vi "detencion.vi"(7 "This VI":refnum<vi>, 8 "error in (no error)":errorcluster, 9 "Air flow":refnum<vi>, 10 "Water flow":refnum<vi>) -> (0 "error out":errorcluster)   [LabVIEW 2013]
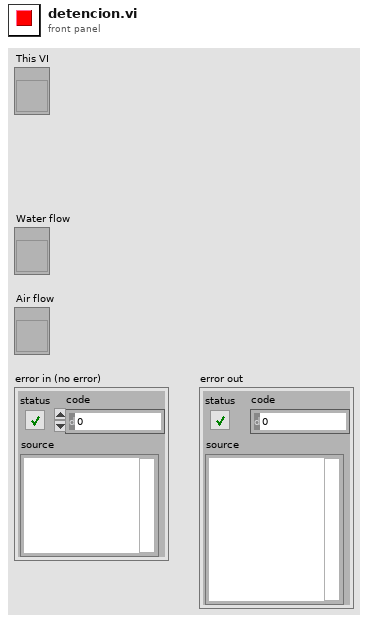
[diagram p1: front panel]
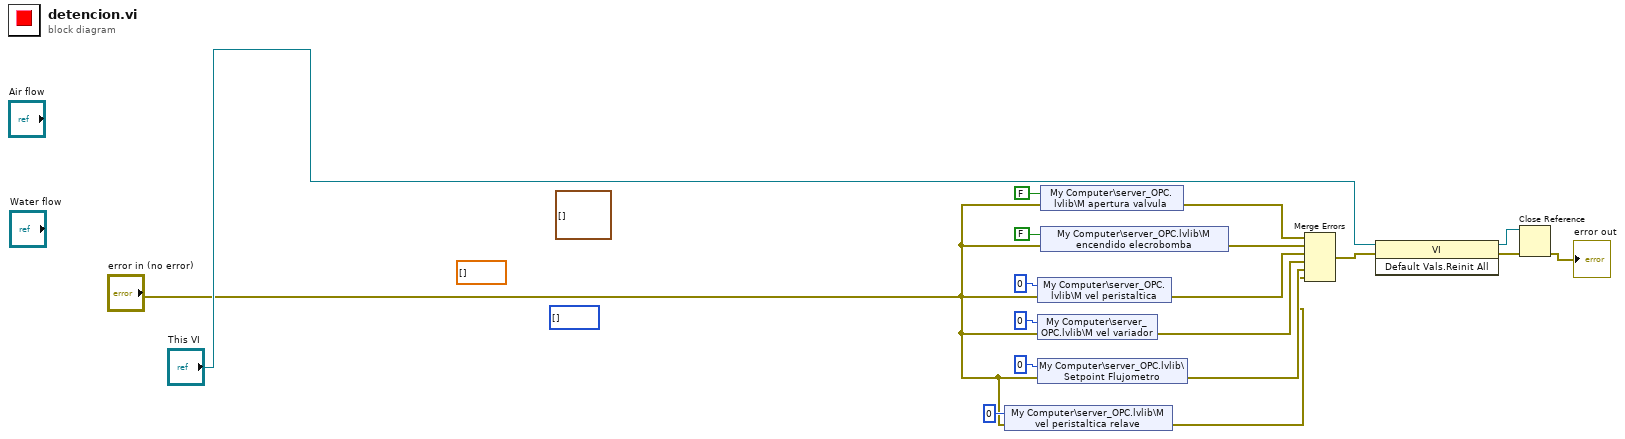
[diagram p0: block diagram]
diagram:
  (unwired) cluster{"pulp flow":dbl, "water flow":dbl}[] [] ("History Data")
  (unwired) dbl[] [] ("History Data")
  (unwired) u16[] [] ("History Data")
  n1 = shared-variable "My Computer\\server_OPC.lvlib\\M vel peristaltica relave"(u16 0 ("M vel peristaltica relave"), error in="error in (no error)") -> (error out=w3:errorcluster)
  n2 = shared-variable "My Computer\\server_OPC.lvlib\\M vel peristaltica"(u16 0 ("M vel peristaltica"), error in="error in (no error)") -> (error out=w9:errorcluster)
  n3 = shared-variable "My Computer\\server_OPC.lvlib\\M vel variador"(u16 0 ("M vel variador"), error in="error in (no error)") -> (error out=w4:errorcluster)
  n4 = shared-variable "My Computer\\server_OPC.lvlib\\Setpoint Flujometro"(u16 0 ("Setpoint Flujometro"), error in="error in (no error)") -> (error out=w10:errorcluster)
  n5 = shared-variable "My Computer\\server_OPC.lvlib\\M apertura valvula"(FALSE ("M apertura valvula"), error in="error in (no error)") -> (error out=w15:errorcluster)
  n6 = shared-variable "My Computer\\server_OPC.lvlib\\M encendido elecrobomba"(FALSE ("M encendido elecrobomba"), error in="error in (no error)") -> (error out=w8:errorcluster)
  n7 = Merge Errors(w15, w8, w9, w4, w10, w3) -> (w16:errorcluster)
  n8 = invoke class="VI" method="Default Vals.Reinit All"(reference="This VI", error in=w16) -> (reference out=w7:refnum<vi>, error out=w6:errorcluster)  [unwired: 1 in, 1 out]
  n9 = Close Reference(reference=w7, error in (no error)=w6) -> (error out=→"error out":errorcluster)
